vi "Payload to String.vi"(8 "error in (no error)":errorcluster, 11 "payload":u8[](array[numeric])=[3, 0, 7, 0, 255]) -> (0 "error out":errorcluster, 3 "Payload String":string)   [LabVIEW 2023]
panel:
  out "Boolean":bool
  out "unsigned byte array":u8[](array[numeric])
  out "string":string
  in  "replace string (\"\")":string
  out "result string":string
  out "x = y?":bool
  in  "y":string
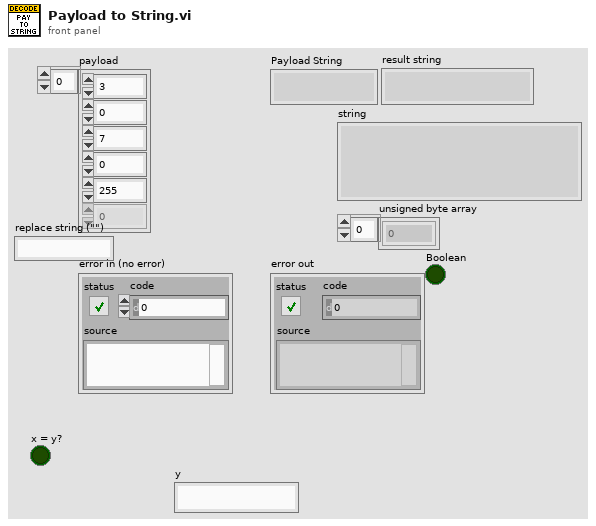
[diagram p1: front panel]
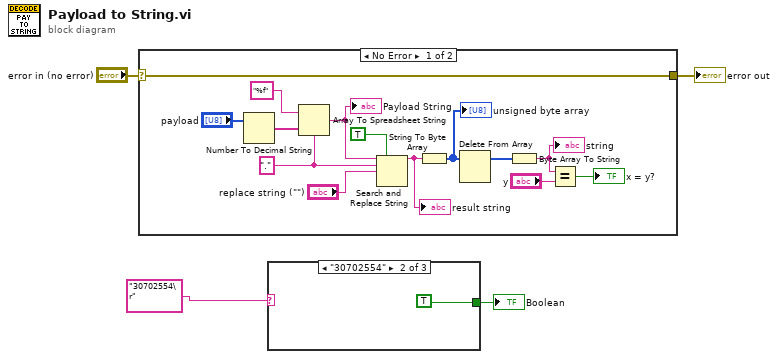
[diagram p0: block diagram]
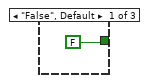
[diagram p2: hidden frame]
diagram:
  n1 = case shown="No Error" "error in (no error)" {
    selector: "error in (no error)" -> [w15 w19]
    tunnel: [w15 w19] -> w3
    frame No Error {
      w10 = "." ("delimiter (Tab)")
      n2 = Number To Decimal String(number="payload") -> (decimal integer string=w17:string[])  [unwired: 1 in]
      n3 = Array To Spreadsheet String(delimiter (Tab)=w10, array=w17, 3:"%f" ("format string")) -> (spreadsheet string=w12:string)
      "Payload String" <- w12
      n4 = Search and Replace String(replace all?=TRUE ("replace all? (F)"), input string=w12, search string=w10, replace string="replace string (\"\")") -> (result string=w8:string)  [unwired: 4 in, 3 out]
      "result string" <- w8
      n5 = String To Byte Array(string=w8) -> (unsigned byte array=w5:u8[])
      "unsigned byte array" <- w5
      n6 = Delete From Array(array=w5) -> (array with subset deleted=w7:u8[])  [unwired: 2 in, 1 out]
      n7 = Byte Array To String(unsigned byte array=w7) -> (string=w6:string)
      "string" <- w6
      n8 = Equal?(x=w6, y="y") -> (x = y?=→"x = y?":bool)
    }
    frame Error {
    }
  }
  "error out" <- w3
  n9 = case shown="\"30702554\"" "30702554\r" {
    tunnel: [FALSE ("Boolean 2") TRUE _] -> w1
    frame "False", Default {
    }
    frame "30702554" {
    }
    frame ? {
    }
  }
  "Boolean" <- w1
